vi "Read Variable (double).vi"(8 "error in (no error)":errorcluster, 9 "Datatype":dbl, 10 "PG path":string, 11 "Data.PGQL in":refnum<class "LV-Data.PGSQL.lvclass">) -> (0 "error out":errorcluster, 1 "Time Stamp":timestamp=timestamp(-9593186400 s since 1904-01-01), 2 "Value":dbl, 3 "Data.PGSQL out":refnum<class "LV-Data.PGSQL.lvclass">)   [LabVIEW 2019, in "LV-Data.PGSQL.lvclass"]
uses:
  LV-Data.PGSQL.lvclass
panel:
  out "Column (units)":string
  out "SQL string":string
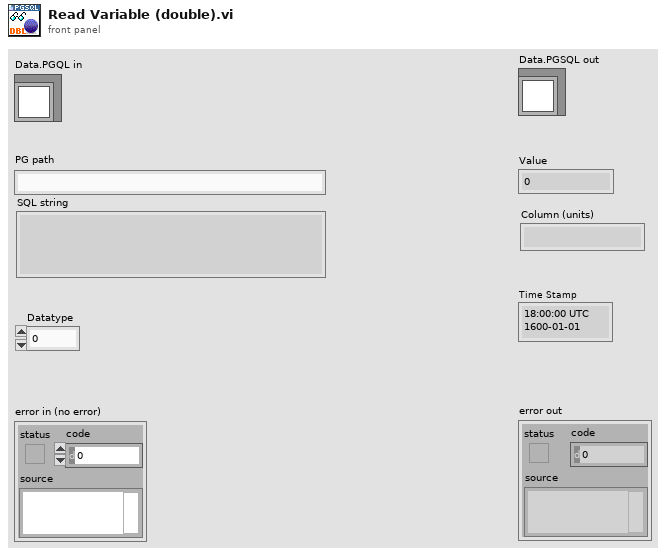
[diagram p1: front panel]
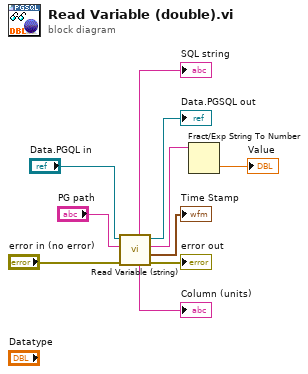
[diagram p0: block diagram]
diagram:
  n1 = call "Read Variable (string).vi"("error in (no error)"="error in (no error)", "PG path"="PG path", "Data.PGQL in"="Data.PGQL in") -> ("error out"=→"error out":errorcluster, "Time Stamp"=→"Time Stamp":timestamp, "Value"=w7:string, "Data.PGSQL out"=→"Data.PGSQL out":refnum<class "LV-Data.PGSQL.lvclass">, "Column (units)"=→"Column (units)":string, "SQL string"=→"SQL string":string)  [unwired: 3 in]
  n2 = Fract/Exp String To Number(string=w7) -> (number=→"Value":dbl)  [unwired: 3 in, 1 out]
